vi "SerialRead.vi"(0 "RIO Device":T1="RIO0", 1 "error in (no error)":errorcluster) -> (2 "RIO Device out":T1, 3 "Serial String":string, 4 "error out":errorcluster)   [LabVIEW 2018]
uses:
  <vilib>/userdefined/High Color/nirio_resource_hc.ctl
panel:
  out "Data ID":u8[](array[numeric]) format="%.0x"
  out "Data":u8[](array[numeric]) format="%.0x"
  out "Progressive":u16=1
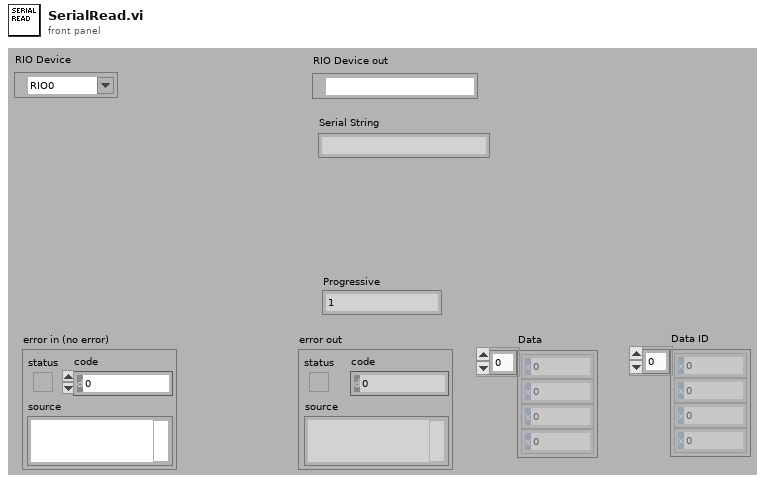
[diagram p1: front panel]
types:
  T1 = typedef "nirio_resource_hc.ctl" = tag
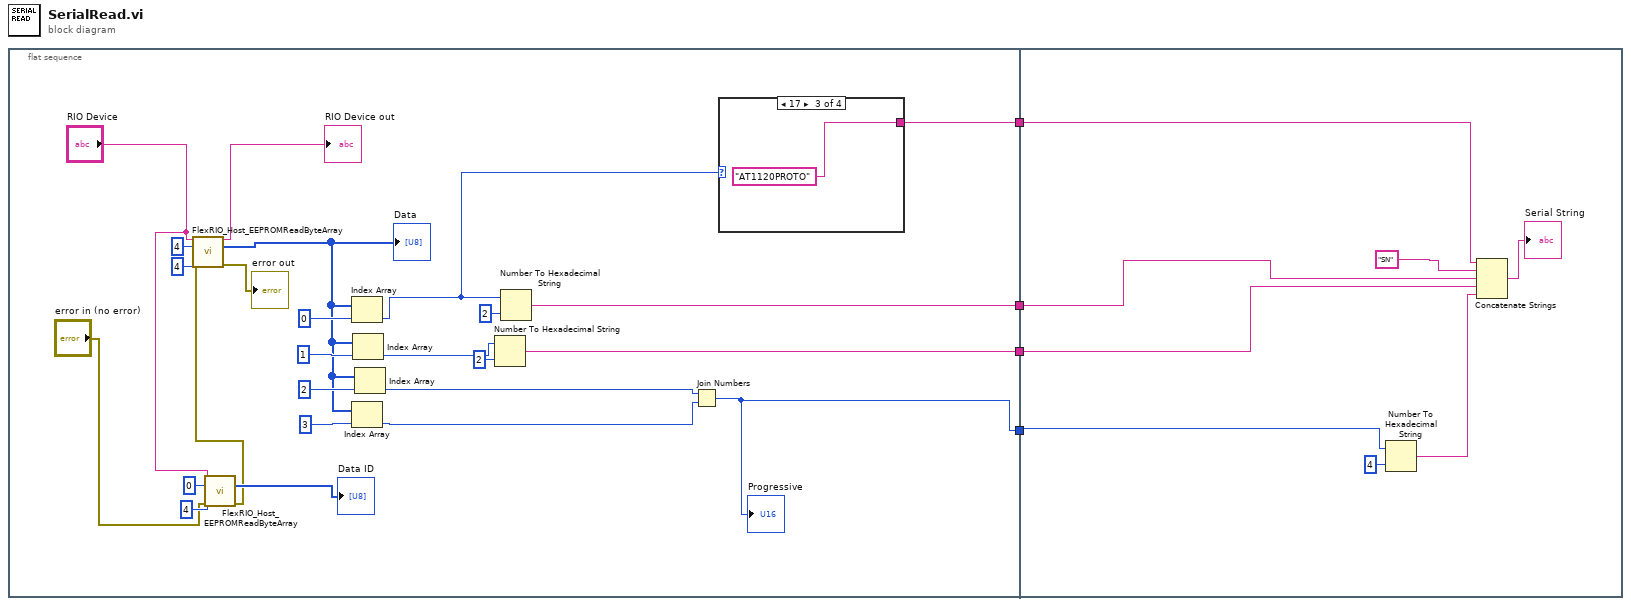
[diagram p0: block diagram]
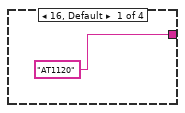
[diagram p2: hidden frame]
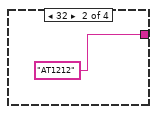
[diagram p3: hidden frame]
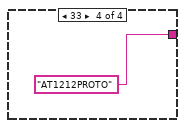
[diagram p4: hidden frame]
diagram:
  n1 = flat-sequence {
    tunnel: [w17] -> w4
    tunnel: [w13] -> w3
    tunnel: [w12] -> w2
    tunnel: [w8] -> w1
    tunnel: w4 -> [w40]
    tunnel: w3 -> [w37]
    tunnel: w2 -> [w36]
    tunnel: w1 -> [w34]
    frame #0 {
      n2 = call <vilib>:"FlexRIO_Host_EEPROMReadByteArray.vi"("RIO Device"="RIO Device", "Address"=u8 0, "Size (bytes)"=u16 4, "error in (no error)"="error in (no error)") -> ("Data"=→"Data ID":u8[], "error out"=w5:errorcluster)  [unwired: 9 in, 1 out]
      n3 = call <vilib>:"FlexRIO_Host_EEPROMReadByteArray.vi"("RIO Device"="RIO Device", "Address"=u8 4, "Size (bytes)"=u16 4, "error in (no error)"=w5) -> ("RIO Device out"=→"RIO Device out":T1, "Data"=w23:u8[], "error out"=→"error out":errorcluster)  [unwired: 9 in]
      "Data" <- w23
      n4 = Index Array(array=w23, index=0) -> (element=w9:u8)
      n5 = Index Array(array=w23, index=3) -> (element=w15:u8)
      n6 = Index Array(array=w23, index=1) -> (element=w14:u8)
      n7 = Index Array(array=w23, index=2) -> (element=w16:u8)
      n8 = Number To Hexadecimal String(1:i16 2 ("width (-)"), 2:w14) -> (0:w12:string)
      n9 = Number To Hexadecimal String(1:i16 2 ("width (-)"), 2:w9) -> (0:w13:string)
      n10 = Join Numbers(hi=w16, lo=w15) -> ((hi.lo)=w17:u16)
      "Progressive" <- w17
      n11 = case shown="17" w9 {
        tunnel: ["AT1120" ("string") "AT1212" ("string") "AT1120PROTO" ("string") "AT1212PROTO" ("string")] -> w8
        frame 16, Default {
        }
        frame 32 {
        }
        frame 17 {
        }
        frame 33 {
        }
      }
    }
    frame #1 {
      n12 = Number To Hexadecimal String(1:i16 4 ("width (-)"), 2:w40) -> (0:w35:string)
      n13 = Concatenate Strings(w34, "SN" ("string"), w37, w36, w35) -> (→"Serial String":string)
    }
  }
